vi "Rectangle Sub-Parser.vi"(3 "error in (no error)":errorcluster, 5 "XML File Path In":path) -> (0 "error out":errorcluster, 1 "rects":T2(array[cluster]), 2 "XML File Path Out":path)   [LabVIEW 2013]
uses:
  <vilib>/Analysis/Matrix/Datatypes/RealMatrix.ctl
  <vilib>/Analysis/baseanly.llb/Real A x B.vi
  <vilib>/Analysis/NI_AALBase.lvlib
  <vilib>/Analysis/Matrix/NI_Matrix.lvlib
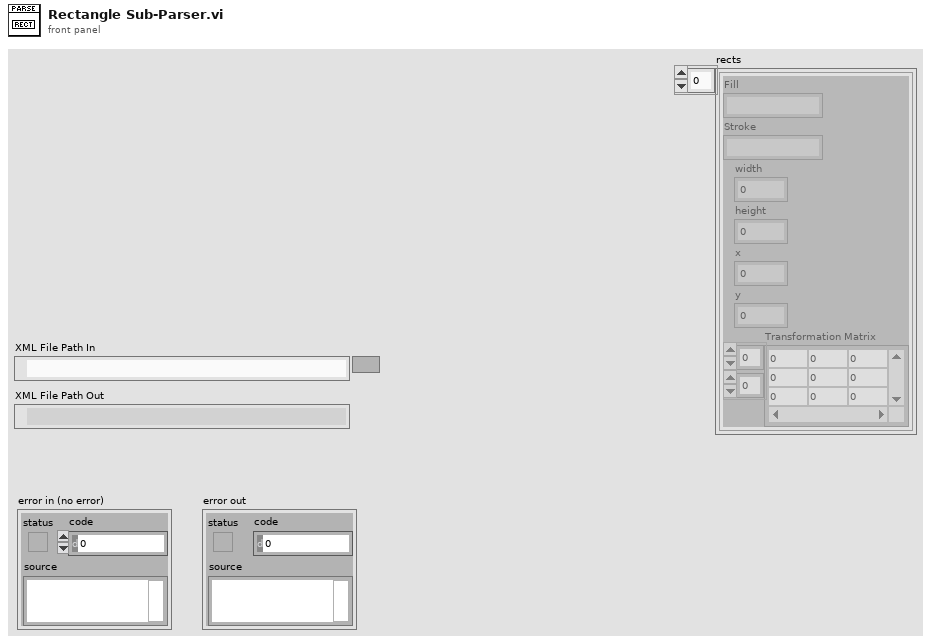
[diagram p1: front panel]
types:
  T1 = typedef "NI_Matrix.lvlib/RealMatrix.ctl" = dbl[][]
  T2 = cluster{"Fill":string, "Stroke":string, "width":dbl, "height":dbl, "x":dbl, "y":dbl, "Transformation Matrix":T1}[]
  T3 = cluster{"Fill":string, "Stroke":string, "Numeric":dbl, "Numeric":dbl, "Numeric":dbl, "Numeric":dbl, "Transformation Matrix":T1}
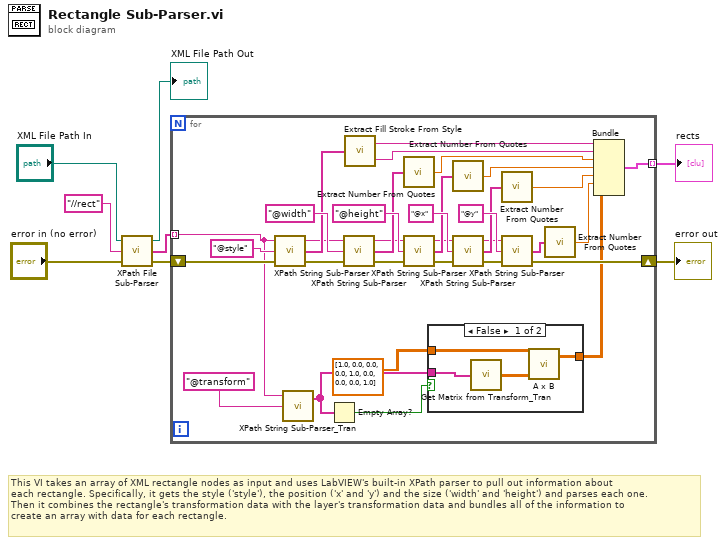
[diagram p0: block diagram]
diagram:
  # "This VI takes an array of XML rectangle nodes as input and uses LabVIEW's built-in XPath parser to pull out information about \neach rectangle. Specifically, it gets the style ('style'), the position ('x' and 'y') and the size ('width' and 'height') and parses each one.\nThen it combines the rectangle's transformation data with the layer's transformation data and bundles all of the information to\ncreate an array with data for each rectangle."
  n1 = call "XPath File Sub-Parser.vi"("error in (no error)"="error in (no error)", "XPath Expression"="//rect" ("XPath expression"), "XML File Path In"="XML File Path In") -> ("error out"=w3:errorcluster, "Array of Results"=w5:string[], "XML File Path Out"=→"XML File Path Out":path)
  n2 = for {
    tunnel: w5 -> [w14] mode=indexing
    shift-right: [w31] -> w8
    shift-left: w3 -> [w39]
    tunnel: [w30] -> w1 mode=indexing
    n3 = call "XPath String Sub-Parser.vi"("error in (no error)"=w39, "XPath expression"="@style", "XML String In"=w14) -> ("error out"=w38:errorcluster, "Array of Results"=w23:string[], "XML String Out"=w18:string)
    n4 = call "XPath String Sub-Parser_Tran.vi"("XPath expression"="@transform", "XML String"=w14) -> ("Array of Results"=w11:string[])  [unwired: 1 in, 1 out]
    n5 = Empty Array?(array=w11) -> (empty?=w12:bool)
    n6 = call "XPath String Sub-Parser.vi"("error in (no error)"=w38, "XPath expression"="@width", "XML String In"=w18) -> ("error out"=w37:errorcluster, "Array of Results"=w22:string[], "XML String Out"=w17:string)
    n7 = call "Extract Fill Stroke From Style.vi"("Array of Results"=w23) -> ("Fill"=w28:string, "Stroke"=w27:string)
    n8 = call "Extract Number From Quotes.vi"("Array of Results"=w22) -> ("Numeric"=w24:dbl)
    n9 = call "XPath String Sub-Parser.vi"("error in (no error)"=w37, "XPath expression"="@height", "XML String In"=w17) -> ("error out"=w36:errorcluster, "Array of Results"=w21:string[], "XML String Out"=w16:string)
    n10 = case shown="False" w12 {
      tunnel: [w45 w46] -> w9
      tunnel: w11 -> [w43 _]
      tunnel: T1 [[1.0, 0.0, 0.0], [0.0, 1.0, 0.0], [0.0, 0.0, 1.0]] ("Transformation Matrix") -> [w42 w46]
      frame False {
        n11 = call "Get Matrix from Transform_Tran.vi"("Transform Attributes"=w43) -> ("Matrix"=w44:T1)
        n12 = call-poly <vilib>:"A x B.vi"("B"=w44, "A"=w42) -> ("A x B"=w45:T1)  [unwired: 1 out]
      }
      frame True {
      }
    }
    n13 = call "Extract Number From Quotes.vi"("Array of Results"=w21) -> ("Numeric"=w29:dbl)
    n14 = call "XPath String Sub-Parser.vi"("error in (no error)"=w36, "XPath expression"="@x", "XML String In"=w16) -> ("error out"=w33:errorcluster, "Array of Results"=w20:string[], "XML String Out"=w15:string)
    n15 = call "Extract Number From Quotes.vi"("Array of Results"=w20) -> ("Numeric"=w25:dbl)
    n16 = call "XPath String Sub-Parser.vi"("error in (no error)"=w33, "XPath expression"="@y", "XML String In"=w15) -> ("error out"=w31:errorcluster, "Array of Results"=w19:string[])  [unwired: 1 out]
    n17 = call "Extract Number From Quotes.vi"("Array of Results"=w19) -> ("Numeric"=w26:dbl)
    n18 = Bundle("Fill"=w28, "Stroke"=w27, "Numeric"=w24, "Numeric"=w29, "Numeric"=w25, "Numeric"=w26, "Transformation Matrix"=w9) -> (w30:T3)  [unwired: 1 in]
  }
  "error out" <- w8
  "rects" <- w1
